vi "Autosort Parameters Set.vi"() -> ()   [LabVIEW 2016]
uses:
  Autosort Parameters.ctl
panel:
  in  "Autosort Parameters Set":T1[](array[typedef])
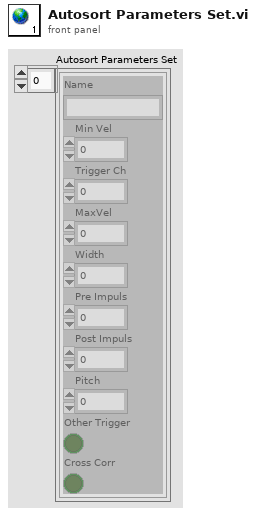
[diagram p1: front panel]
types:
  T1 = typedef "Autosort Parameters.ctl" = cluster{"Name":string, "Min Vel":dbl, "Trigger Ch":i32, "MaxVel":dbl, "Width":i32, "Pre Impuls":i32, "Post Impuls":i32, "Pitch":dbl, "Other Trigger":bool, "Cross Corr":bool}
diagram:
